vi "Light Close.vi"(8 "error in (no error)":errorcluster, 11 "Lighting Refnum In":refnum<k1>) -> (0 "error out":errorcluster)   [LabVIEW 2010]
doc: "Closes the Theatre Lighting Hardware Device."
uses:
  Refnum Enum.ctl
panel:
  # "Input Data"
  # "Local Data"
  # "Output Data"
  # "No Local Data"
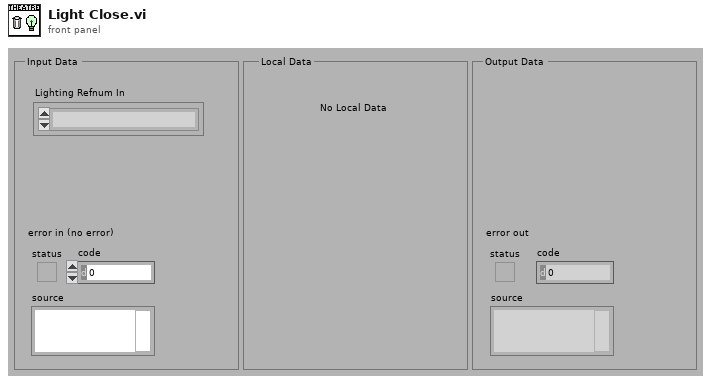
[diagram p1: front panel]
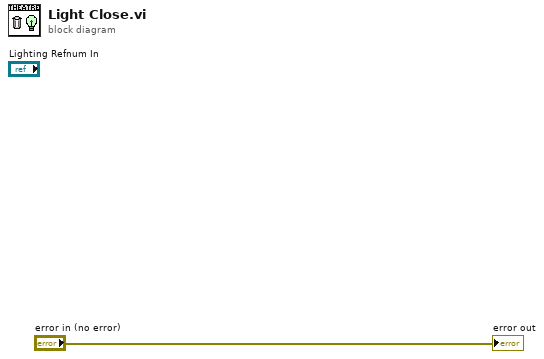
[diagram p0: block diagram]
diagram:
  "error out" <- "error in (no error)"
